vi "Register gRPC Methods.vi"(8 "error in":errorcluster, 11 "gRPC service in":refnum<class "ServiceBase.lvclass">) -> (0 "error out":errorcluster, 3 "gRPC service out":refnum<class "ServiceBase.lvclass">)   [LabVIEW 2019, in "gRPC-servicer.lvlib" / "ServiceBase.lvclass"]
uses:
  ServiceBase.lvclass
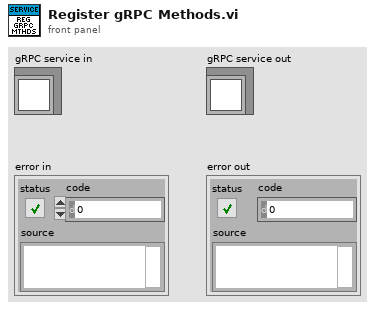
[diagram p1: front panel]
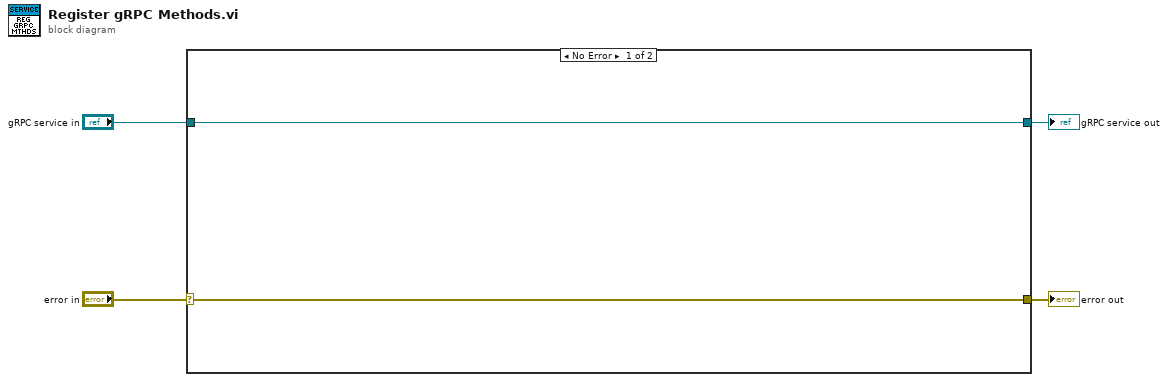
[diagram p0: block diagram]
diagram:
  n1 = case shown="No Error" "error in" {
    selector: "error in" -> [w6 w8]
    tunnel: "gRPC service in" -> [w5 w7]
    tunnel: [w6 w8] -> w4
    tunnel: [w5 w7] -> w1
    frame No Error {
    }
    frame Error {
    }
  }
  "error out" <- w4
  "gRPC service out" <- w1
